vi "Set trigger.vi"(8 "error in (no error)":errorcluster, 11 "DAQOrcaFlash in":refnum<class "DAQOrcaFlash.lvclass">) -> (0 "error out":errorcluster, 3 "DAQOrcaFlash out":refnum<class "DAQOrcaFlash.lvclass">)   [LabVIEW 2012, in "DAQOrcaFlash.lvclass"]
uses:
  DAQOrcaFlash.lvclass
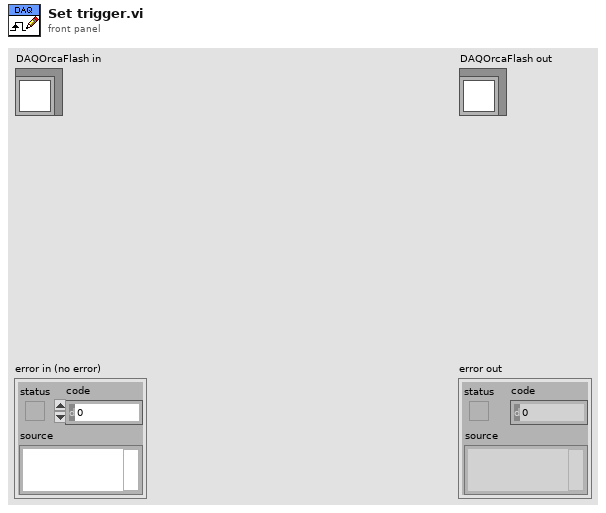
[diagram p1: front panel]
types:
  T1 = typedef "DAQOrcaFlash.lvclass/trigger_mode.ctl" = sgl
  T2 = typedef "DAQOrcaFlash.lvclass/trigger_source.ctl" = sgl
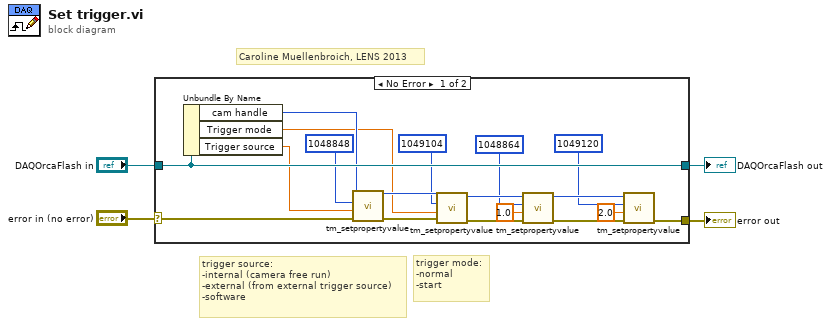
[diagram p0: block diagram]
diagram:
  # "trigger mode:\n-normal\n-start"
  # "trigger source:\n-internal (camera free run) \n-external (from external trigger source)\n-software"
  # "Caroline Muellenbroich, LENS 2013"
  n1 = case shown="No Error" "error in (no error)" {
    selector: "error in (no error)" -> [w17 w24]
    tunnel: [w11 w24] -> w3
    tunnel: [w22 w23] -> w1
    tunnel: "DAQOrcaFlash in" -> [w22 w23]
    frame No Error {
      n2 = Unbundle By Name(w22) -> ("cam handle"=w21:u32, "Trigger mode"=w14:T1, "Trigger source"=w15:T2)
      n3 = call <userlib>:"tm_setpropertyvalue.vi"("error in (no error)"=w17, "Value in"=w15, "Property ID"=u32 1048848, "Handle in"=w21) -> ("error out"=w16:errorcluster, "Handle out"=w20:u32)  [unwired: 6 in]
      n4 = call <userlib>:"tm_setpropertyvalue.vi"("error in (no error)"=w16, "Value in"=w14, "Property ID"=u32 1049104, "Handle in"=w20) -> ("error out"=w13:errorcluster, "Handle out"=w10:u32)  [unwired: 6 in]
      n5 = call <userlib>:"tm_setpropertyvalue.vi"("error in (no error)"=w13, "Value in"=sgl 1.0, "Property ID"=u32 1048864, "Handle in"=w10) -> ("error out"=w12:errorcluster, "Handle out"=w9:u32)  [unwired: 6 in]
      n6 = call <userlib>:"tm_setpropertyvalue.vi"("error in (no error)"=w12, "Value in"=sgl 2.0, "Property ID"=u32 1049120, "Handle in"=w9) -> ("error out"=w11:errorcluster)  [unwired: 6 in, 1 out]
    }
    frame Error {
    }
  }
  "error out" <- w3
  "DAQOrcaFlash out" <- w1
